vi "配置文件保存.vi"   [LabVIEW 2016, in "斯坦道多参数.lvlib"]
uses:
  <vilib>/Utility/config.llb/NI_LVConfig.lvlib
types:
  T1 = typedef "NI_LVConfig.lvlib/Config Data RefNum.ctl" = refnum<k1>
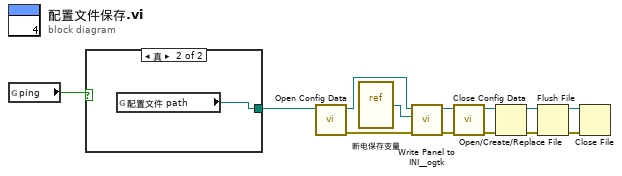
[diagram p0: block diagram]
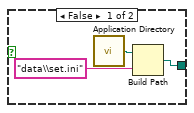
[diagram p2: hidden frame]
diagram:
  n1 = global read "多参数全局变量.vi" "ping"() -> (w2:bool)
  n2 = case shown="真" w2 {
    tunnel: [w14 w17] -> w1
    frame False {
      n3 = call <vilib>:"Application Directory.vi"() -> ("Application Directory"=w15:path)
      n4 = Build Path(base path=w15, name or relative path="data\\set.ini" ("名称或相对路径")) -> (appended path=w14:path)
    }
    frame True {
      n5 = global read "多参数全局变量.vi" "配置文件 path"() -> (w17:path)
    }
  }
  n6 = call <vilib>:"Open Config Data.vi"("configuration file path"=w1) -> ("error out"=w12:errorcluster, "refnum"=w13:T1)  [unwired: 8 in, 1 out]
  n7 = vi-ref "断电保存变量.vi"() -> (w9:refnum<vi>)
  n8 = call <userlib>:"Write Panel to INI__ogtk.vi"("error in (no error)"=w12, "VI ref"=w9, "refnum"=w13) -> ("error out"=w10:errorcluster, "refnum out"=w11:T1)  [unwired: 7 in]
  n9 = call <vilib>:"Close Config Data.vi"("error in (no error)"=w10, "refnum"=w11) -> ("error out"=w5:errorcluster, "file path"=w6:path)  [unwired: 8 in]
  n10 = Open/Create/Replace File(file path (use dialog)=w6, error in=w5) -> (refnum out=w7:refnum<file>, error out=w8:errorcluster)  [unwired: 4 in, 1 out]
  n11 = Flush File(refnum=w7, error in=w8) -> (refnum out=w3:refnum<file>, error out=w4:errorcluster)
  n12 = Close File(refnum=w3, error in=w4) -> ()  [unwired: 2 out]
